vi "Command 7265.vi"(8 "error in (no error)":errorcluster, 10 "Command":string="OF. 11.113", 11 "7265 GPIB":string="7") -> (0 "error out":errorcluster)   [LabVIEW 2013]
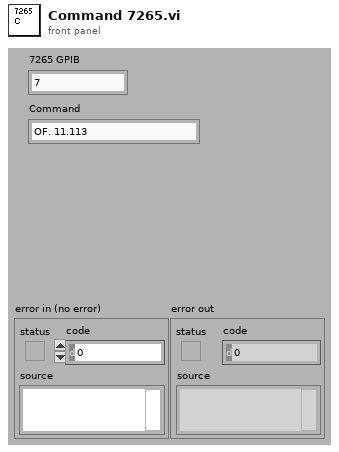
[diagram p1: front panel]
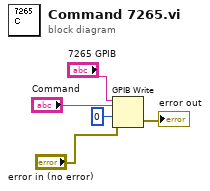
[diagram p0: block diagram]
diagram:
  n1 = GPIB Write(0:"7265 GPIB", 1:"Command", 2:i16 0 ("mode (0)"), 3:"error in (no error)") -> (6:→"error out":errorcluster)  [unwired: 1 in, 1 out]
